vi "Loss测量.vi"(7 "VISA resource name":refnum<visa-resource-name>, 8 "error in (no error)":errorcluster, 10 "Freq":dbl[](array[numeric]), 11 "network in":refnum<class "network.lvclass">) -> (0 "error out":errorcluster, 1 "S12":dbl[](array[numeric]), 2 "S11":dbl[](array[numeric]), 3 "network out":refnum<class "network.lvclass">, 4 "S22":dbl[](array[numeric]), 5 "freq":dbl[](array[numeric]), 6 "S21":dbl[](array[numeric]))   [LabVIEW 2015, in "network.lvclass"]
uses:
  network.lvclass
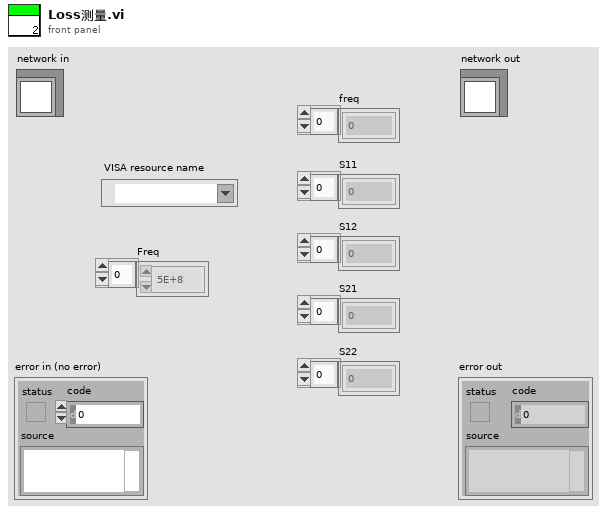
[diagram p1: front panel]
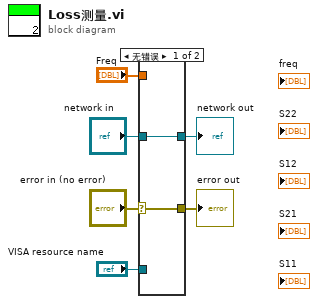
[diagram p0: block diagram]
diagram:
  n1 = case shown="无错误" "error in (no error)" {
    selector: "error in (no error)" -> [w7 w10]
    tunnel: [w7 w10] -> w5
    tunnel: [w8 w9] -> w3
    tunnel: "network in" -> [w8 w9]
    tunnel: "VISA resource name" -> [_ _]
    tunnel: "Freq" -> [_ _]
    frame No Error {
    }
    frame Error {
    }
  }
  "error out" <- w5
  "network out" <- w3
